vi "xiLIB - LoadFromINI_DIALOG.vi"(6 "IniPath":path=path "C:/Users/Durnek60/Desktop/3DLIB/APP_REQ/APP_FOLDER/Setup/Param.ini", 8 "error in (no error)":errorcluster, 11 "xiCam In":refnum<k24>) -> (0 "error out":errorcluster={"status"=TRUE, "code"=-1, "source"="Parameter file not found at location: \n\nC:\\Users\\Durnek60\\Desktop\\3DLIB\\Resources\\Cam_PRM.ini"}, 3 "xiCam Out":refnum<k24>)   [LabVIEW 2018]
doc: "Dialog based parameter load function."
uses:
  D:/codes labview/VisionLibrariesXimea/xiLib/xiLIB_64bit/xiLIB/xiCamLib/API/x64/xiApi.NETX64.dll
  API/x64/xiApi.NETX64.dll
  xiCam/PRM/PRM/PRM_v2.ctl
  <vilib>/Utility/miscctls.llb/LVRowAndColumnTypeDef.ctl
  <vilib>/Utility/config.llb/NI_LVConfig.lvlib
panel:
  in  "MCL":i32(listbox)=-1
  out "Slide":i32(slide) caption="Loading..." min=0 scale=0.0..91.0
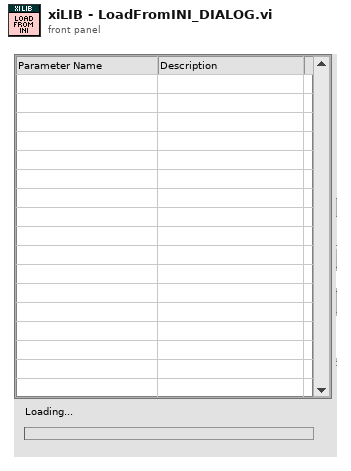
[diagram p1: front panel]
types:
  T1 = typedef "PRM_v2.ctl" = enum16{"ACQ_BUFFER_SIZE", "ACQ_FRAME_BURST_COUNT", "ACQ_TIMING_MODE", "ACQ_TRANSPORT_BUFFER_SIZE", "AE_MAX_LIMIT", "AEAG", "AEAG_LEVEL", "API_VERSION", "AG_MAX_LIMIT", "APPLY_CMS", "AUTO_BANDWIDTH_CALCULATION", "AUTO_WB", "AVAILABLE_BANDWIDTH", "AVAILABLE_BANDWIDTH_MAX", "AVAILABLE_BANDWIDTH_MIN", "BPC", "BUFFER_POLICY", "BUFFERS_QUEUE_SIZE", "CC_MATRIX_00", "CC_MATRIX_01", "CC_MATRIX_02", "CC_MATRIX_03", "CC_MATRIX_10", "CC_MATRIX_11", "CC_MATRIX_12", "CC_MATRIX_13", "CC_MATRIX_20", "CC_MATRIX_21", "CC_MATRIX_22", "CC_MATRIX_23", "CC_MATRIX_30", "CC_MATRIX_31", "CC_MATRIX_32", "CC_MATRIX_33", "CHIP_TEMP", "CMS", "COLOR_FILTER_ARRAY", "COOLING", "DEBOUNCE_EN", "DEBOUNCE_POL", "DEBOUNCE_T0", "DEBOUNCE_T1", "DEBUG_LEVEL", "DEFAULT_CC_MATRIX", "DEVICE_INSTANCE_PATH", "DEVICE_MODEL_ID", "DEVICE_NAME", "DEVICE_SN", "DEVICE_TYPE", "DEVICE_USER_ID", "DOWNSAMPLING", "DOWNSAMPLING_MAX", "DOWNSAMPLING_MIN", "DOWNSAMPLING_TYPE", "DRV_VERSION", "EXP_PRIORITY", "EXPOSURE", "EXPOSURE_DIRECT_UPDATE", "EXPOSURE_MAX", "EXPOSURE_MIN", "FFS_FILE_NAME", "FPGA1_VERSION", "FRAMERATE", "FRAMERATE_MAX", "FRAMERATE_MIN", "FREE_FFS_SIZE", "GAIN", "GAIN_DIRECT_UPDATE", "GAIN_MAX", "GAIN_MIN", "GAMMAC", "GAMMAY", "GPI_LEVEL", "GPI_MODE", "GPI_SELECTOR", "GPI_SELECTOR_MAX", "GPI_SELECTOR_MIN", "GPO_MODE", "GPO_SELECTOR", "GPO_SELECTOR_MAX", "GPO_SELECTOR_MIN", "HDR", "HDR_T1", "HDR_T2", "HEIGHT", "HEIGHT_MAX", "HEIGHT_MIN", "HOUSE_TEMP", "IMAGE_DATA_FORMAT", "IMAGE_IS_COLOR", "INPUT_CMS_PROFILE", "IS_COOLED", "IS_DEVICE_EXIST", "KNEEPOINT1", "KNEEPOINT2", "LED_MODE", "LED_SELECTOR", "LED_SELECTOR_MAX", "LED_SELECTOR_MIN", "LIMIT_BANDWIDTH", "LIMIT_BANDWIDTH_MAX", "LIMIT_BANDWIDTH_MIN", "LUT_EN", "LUT_INDEX", "LUT_INDEX_MAX", "LUT_INDEX_MIN", "LUT_VALUE", "LUT_VALUE_MAX", "LUT_VALUE_MIN", "MANUAL_WB", "MCU1_VERSION", "MCU2_VERSION", "OFFSET_X", "OFFSET_X_MAX", "OFFSET_X_MIN", "OFFSET_Y", "OFFSET_Y_MAX", "OFFSET_Y_MIN", "OUTPUT_CMS_PROFILE", "OUTPUT_DATA_BIT_DEPTH", "OUTPUT_DATA_PACKING", "READ_FILE_FFS", "RECENT_FRAME", "SENSOR_DATA_BIT_DEPTH", "SENSOR_MODE", "SENSOR_TAPS", "SHARPNESS", "SHUTTER_TYPE", "TARGET_TEMP", "TRG_DELAY", "TRG_SELECTOR", "TRG_SOFTWARE", "TRG_SOURCE", "USED_FFS_SIZE", "WB_KB", "WB_KG", "WB_KR", "WIDTH", "WIDTH_MAX", "WIDTH_MIN", "WRITE_FILE_FFS", "ACQ_BUFFER_SIZE_UNIT", "ACQ_TRANSPORT_BUFFER_COMMIT", "AEAG_ROI_HEIGHT", "AEAG_ROI_OFFSET_X", "AEAG_ROU_OFFSET_Y", "AEAG_ROI_WIDTH", "API_CONTEXT_LIST", "BINNING_HORIZONTAL", "BINNING_SELECTOR", "BINNING_VERTICAL", "COLUMN_FPN_CORRECTION", "COUNTER_SELECTOR", "COUNTER_VALUE", "DECIMATION_HORIZONTAL", "DECIMATION_SELECTOR", "DECIMATION_VERTICAL", "DEVICE_ID", "DEVICE_LOCATION_PATH", "DEVICE_MANIFEST", "DEVICE_RESET", "DEVICE_SENS_SN", "EXPOSURE_BURST_COUNT", "FFS_ACCESS_KEY", "GAIN_SELECTOR", "HW_REVISION", "IMAGE_BLACK_LEVEL", "IMAGE_DATA_BIT_DEPTH", "IMAGE_DATA_FORMAT_RGB32_ALPHA", "IMAGE_PAYLOAD_SIZE", "LENS_APERTURE_VALUE", "LENS_FEATURE", "LENS_FEATURE_SELECTOR", "LENS_FOCAL_LENGTH", "LENS_FOCUS_DISTANCE", "LENS_FOCUS_MOVE", "LENS_FOCUS_MOVEMENT_VALUE", "LENS_MODE", "OUTPUT_DATA_PACKING_TYPE", "SENSOR_CLOCK_FREQ_HZ", "SENSOR_CLOCK_FREQ_INDEX", "SENSOR_FEATURE_SELECTOR", "SENSOR_FEATURE_VALUE", "SENSOR_OUTPUT_CHANNEL_COUNT", "TRANSPORT_PIXEL_FORMAT", "TS_RST_MODE", "TS_RST_SOURCE"}
  T2 = typedef "LVRowAndColumnTypeDef.ctl" = cluster{"Row":i32, "Column":i32}
  T3 = typedef "NI_LVConfig.lvlib/Config Data RefNum.ctl" = refnum<k1>
  T4 = typedef "xiLIB - PRM_Load_Result.ctl" = enum16{"SUCCESS", "ERROR", "WARNING - Not Valid Parameter", "WARNING - Get Parameter"}
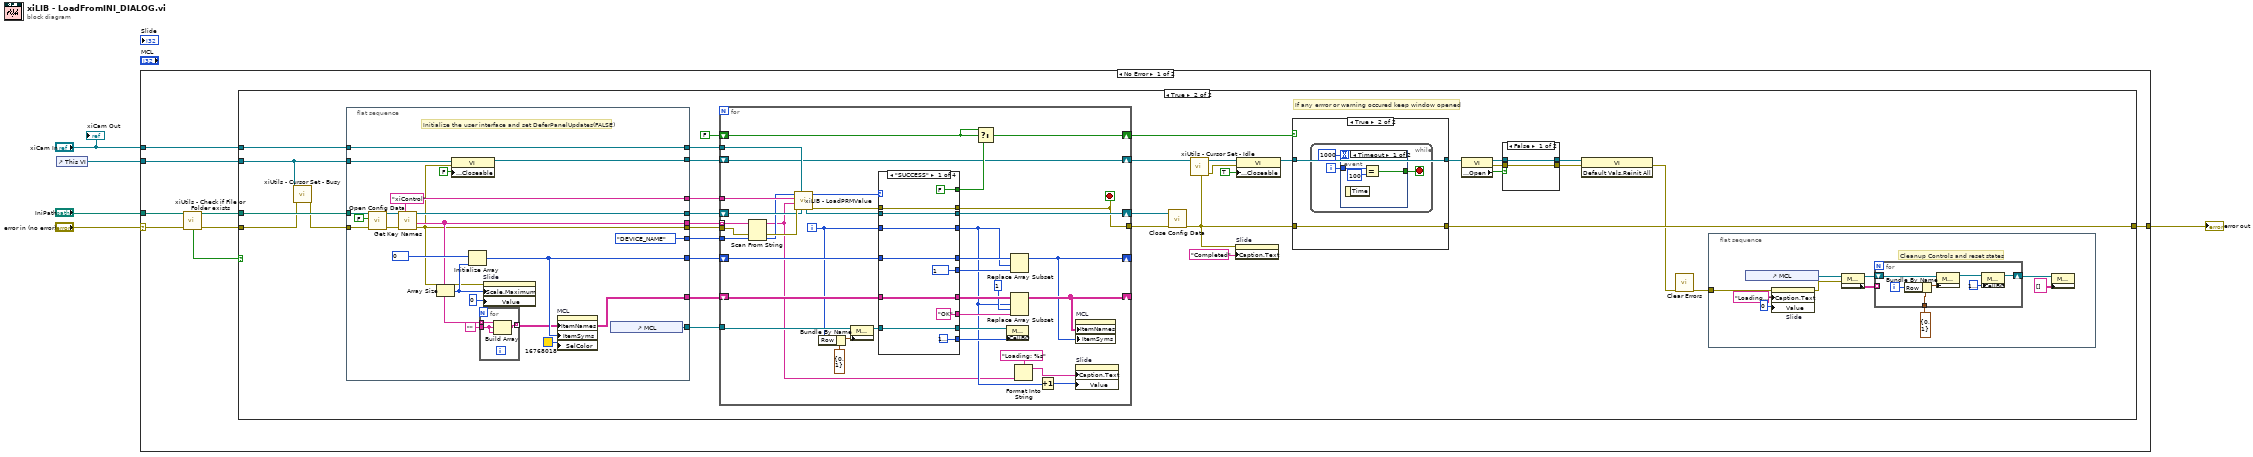
[diagram p0: block diagram]
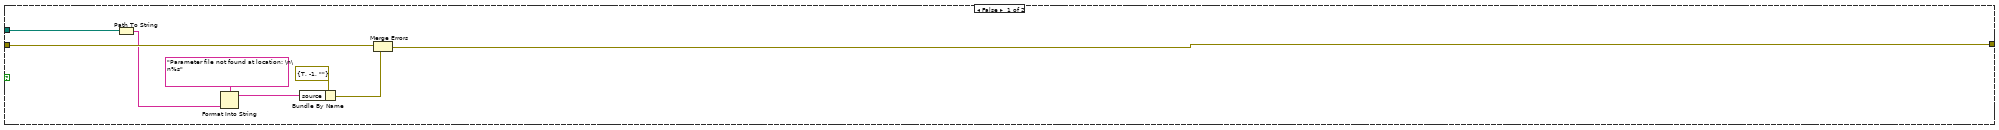
[diagram p2: hidden frame]
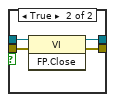
[diagram p3: hidden frame]
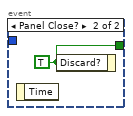
[diagram p5: hidden frame]
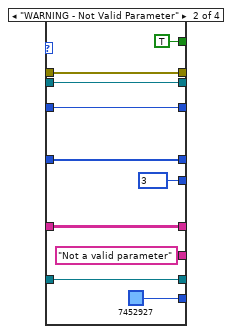
[diagram p6: hidden frame]
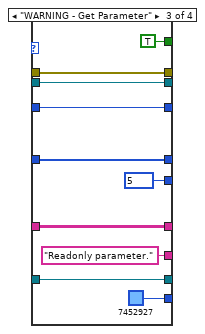
[diagram p7: hidden frame]
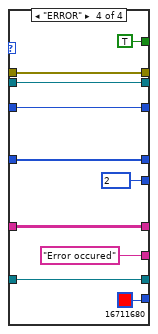
[diagram p8: hidden frame]
diagram:
  n1 = control-ref of="This VI"() -> (w1:refnum<vi>)
  n2 = case shown="No Error" "error in (no error)" {
    selector: "error in (no error)" -> [w10 w192]
    tunnel: [w13 w192] -> w4
    tunnel: "IniPath" -> [w11 _]
    tunnel: "xiCam In" -> [w12 _]
    tunnel: w1 -> [w6 _]
    frame No Error {
      n3 = call "xiUtils - Check if File or Folder exists.vi"("error in (no error)"=w10, "path"=w11) -> ("error out"=w9:errorcluster, "file or folder exists?"=w7:bool, "dup path"=w8:path)  [unwired: 7 in]
      n4 = case shown="True" w7 {
        tunnel: [w20 w44] -> w13
        tunnel: w12 -> [_ w40]
        tunnel: w9 -> [w21 w36]
        tunnel: w8 -> [w19 w38]
        tunnel: w6 -> [_ w37]
        frame False {
          n5 = Path To String(path=w19) -> (string=w17:string)
          n6 = Format Into String(format string="Parameter file not found at location: \n\n%s" ("source"), w17) -> (resulting string=w15:string)  [unwired: 2 in, 1 out]
          n7 = Bundle By Name(cluster=errorcluster {"status"=TRUE, "code"=-1, "source"=""} ("error in"), "source"=w15) -> (w14:errorcluster)
          n8 = Merge Errors(w21, w14) -> (w20:errorcluster)
        }
        frame True {
          # "If any errror or warning occured keep window opened"
          n9 = call "xiUtils - Cursor Set - Busy.vi"("error in (no error)"=w36, "VI reference (Top Level VI)"=w37) -> ("error out"=w35:errorcluster)  [unwired: 8 in, 1 out]
          n10 = flat-sequence {
            tunnel: w38 -> [w83]
            tunnel: w35 -> [w81]
            tunnel: [w78] -> w55
            tunnel: [PRM_v2."DEVICE_NAME" ("PRM")] -> w54
            tunnel: [w76] -> w53
            tunnel: [w71] -> w49
            tunnel: [w70] -> w48
            tunnel: [w68] -> w47
            tunnel: [w67] -> w46
            tunnel: [w66] -> w45
            tunnel: w40 -> [w65]
            tunnel: [w65] -> w39
            tunnel: w37 -> [w63]
            tunnel: [w62] -> w33
            frame #0 {
              w76 = "xiControl" ("section")
              # "Initialize the user interface and set DeferPanelUpdates(FALSE)"
              n11 = call <vilib>:"Open Config Data.vi"("error in (no error)"=w81, "create file if necessary (T)"=FALSE, "configuration file path"=w83) -> ("error out"=w79:errorcluster, "refnum"=w80:T3)  [unwired: 6 in, 1 out]
              n12 = call <vilib>:"Get Key Names.vi"("section"=w76, "error in (no error)"=w79, "refnum"=w80) -> ("error out"=w67:errorcluster, "key names"=w71:string[], "refnum out"=w78:T3)  [unwired: 5 in, 1 out]
              n13 = Array Size(array=w71) -> (size(s)=w72:i32)
              n14 = property class="VI"(reference=w63, error in=w67, "Front Panel.Closeable"=FALSE ("Front Panel Window:Closeable")) -> (reference out=w62:refnum<vi>)  [unwired: 1 out]
              n15 = Initialize Array(0, w72) -> (w70:i32[])
              n16 = for {
                tunnel: w71 -> [w86] mode=indexing
                tunnel: [w85] -> w68 mode=indexing
                tunnel: "" -> [w84]
                n17 = Build Array(w86, w84, w84) -> (w85:string[])
              }
              n18 = property on="Slide" class="Slide (strict)"(error in=w67, "Scale.Maximum"=w72, "Value"=0 ("Slide")) -> ()  [unwired: 1 in, 2 out]
              n19 = property on="MCL" class="MCListbox (strict)"("ItemNames"=w68, "ItemSyms"=w70, "SelColor"=u32 16768018) -> ()  [unwired: 2 in, 2 out]
              n20 = control-ref of="MCL"() -> (w66:refnum<vi>)
            }
          }
          n21 = for {
            shift-right: [w139] -> w52
            shift-left: w55 -> [w149]
            tunnel: w49 -> [w117] mode=indexing
            tunnel: w54 -> [w151]
            tunnel: w46 -> [w148]
            tunnel: w53 -> [w147]
            shift-right: [w122] -> _
            shift-left: w48 -> [w138]
            tunnel: w39 -> [w143]
            shift-right: [w145] -> w50
            shift-left: FALSE -> [w146]
            shift-right: [w123] -> _
            shift-left: w47 -> [w135]
            tunnel: w45 -> [w129]
            tunnel: [w124] -> w42
            shift-right: [w115] -> w32
            shift-left: w33 -> [w115]
            i -> [w128]
            stop <- w124 stop-if-true
            n22 = Scan From String(input string=w117, error in=w148, default 1=w151) -> (error out=w150:errorcluster, output 1=w144:T1)  [unwired: 2 in, 2 out]
            n23 = call "xiLIB - LoadPRMValue.vi"("INI Refnum"=w149, "xiCam In"=w143, "error in (no error)"=w150, "key"=w117, "section"=w147, "PRM"=w144) -> ("error out"=w141:errorcluster, "Load_Result"=w142:T4, "INI Refnum out"=w140:T3)  [unwired: 3 in]
            n24 = Bundle By Name(cluster=T2 {"Row"=0, "Column"=1} ("Active Cell:Active Cell"), "Row"=w128) -> (w130:T2)
            n25 = property class="MCListbox (strict)"(reference=w129, "ActiveCell"=w130) -> (reference out=w127:refnum<vi>)  [unwired: 1 in, 1 out]
            n26 = case shown="\"SUCCESS\"" w142 {
              tunnel: w141 -> [w160 w170 w180 w190]
              tunnel: w140 -> [w161 w171 w181 w191]
              tunnel: [w161 w171 w181 w191] -> w139
              tunnel: [w160 w170 w180 w190] -> w124
              tunnel: w128 -> [w157 w167 w177 w187]
              tunnel: w138 -> [w159 w169 w179 w189]
              tunnel: [w159 w169 w179 w189] -> w137
              tunnel: [1 3 5 2] -> w136
              tunnel: [w157 w167 w177 w187] -> w118
              tunnel: w135 -> [w156 w166 w176 w186]
              tunnel: [w156 w166 w176 w186] -> w134
              tunnel: ["OK" "Not a valid parameter" "Readonly parameter." "Error occured"] -> w132
              tunnel: w127 -> [w155 w164 w173 w184]
              tunnel: [w155 w164 w173 w184] -> w126
              tunnel: [u32 16777233 ("Color Box") u32 7452927 u32 7452927 u32 16711680] -> w125
              tunnel: [FALSE TRUE TRUE TRUE] -> w116
              frame "SUCCESS" {
              }
              frame "WARNING - Not Valid Parameter" {
              }
              frame "WARNING - Get Parameter" {
              }
              frame "ERROR" {
              }
            }
            n27 = Select(t=w146, s=w146, f=w116) -> (s? t:f=w145:bool)
            n28 = property class="MCListbox (strict)"(reference=w126, "CellBG"=w125) -> ()  [unwired: 1 in, 2 out]
            n29 = Replace Array Subset(array=w137, new element=w136, index=w118) -> (w122:i32[])
            n30 = Replace Array Subset(array=w134, new element=w132, index (row)=w118, index (col)=1) -> (w123:string[][])
            n31 = Format Into String(format string="Loading: %s", w117) -> (resulting string=w119:string)  [unwired: 2 in, 1 out]
            n32 = Increment(x=w118) -> (x+1=w121:i32)
            n33 = property on="Slide" class="Slide (strict)"("Caption.Text"=w119, "Value"=w121) -> ()  [unwired: 2 in, 2 out]
            n34 = property on="MCL" class="MCListbox (strict)"("ItemNames"=w123, "ItemSyms"=w122) -> ()  [unwired: 2 in, 2 out]
          }
          n35 = call <vilib>:"Close Config Data.vi"("error in (no error)"=w42, "refnum"=w52) -> ("error out"=w31:errorcluster)  [unwired: 8 in, 1 out]
          n36 = call "xiUtils - Cursor Set - Idle.vi"("error in (no error)"=w31, "VI reference (Top Level VI)"=w32) -> ("error out"=w30:errorcluster)  [unwired: 9 in]
          n37 = property on="Slide" class="Slide (strict)"(error in=w31, "Caption.Text"="Completed" ("format string")) -> ()  [unwired: 1 in, 2 out]
          n38 = property class="VI"(reference=w32, error in=w30, "Front Panel.Closeable"=TRUE ("Front Panel Window:Closeable")) -> (reference out=w26:refnum<vi>)  [unwired: 1 out]
          n39 = case shown="True" w50 {
            tunnel: w31 -> [w105 w107]
            tunnel: [w105 w107] -> w44
            tunnel: w26 -> [w104 w106]
            tunnel: [w104 w106] -> w25
            frame False {
              # "Do nothing, every parameter loaded"
            }
            frame True {
              n40 = while {
                i -> [w108]
                stop <- w110 stop-if-true
                n41 = event shown="[0] Timeout" {
                  selector: _ -> [_ _]
                  dyn-events: _ -> [_ _]
                  timeout: 1000 -> [_ _]
                  tunnel: [w111 w114] -> w110
                  tunnel: w108 -> [w113 _]
                  event Timeout {
                    n42 = event-data() -> ()  [unwired: 1 in, 1 out]
                    n43 = Equal?(x=w113, y=100) -> (x = y?=w111:bool)
                  }
                  event Panel Close? {
                    w114 = TRUE
                    n44 = event-data() -> ()  [unwired: 1 in, 1 out]
                    n45 = event-data("Discard?"=w114) -> ()  [unwired: 1 in, 1 out]
                  }
                }
              }
            }
          }
          n46 = property class="VI"(reference=w25) -> (reference out=w28:refnum<vi>, error out=w29:errorcluster, "Front Panel.Open"=w27:bool)  [unwired: 1 in]
          n47 = case shown="False" w27 {
            tunnel: [w57 w61] -> w23
            tunnel: w29 -> [w57 w60]
            tunnel: w28 -> [w56 w59]
            tunnel: [w56 w58] -> w24
            frame False {
            }
            frame True {
              n48 = invoke class="VI" method="FP.Close"(reference=w59, error in=w60) -> (reference out=w58:refnum<vi>, error out=w61:errorcluster)  [unwired: 1 in, 1 out]
            }
          }
          n49 = invoke class="VI" method="Default Vals.Reinit All"(reference=w24, error in=w23) -> (error out=w22:errorcluster)  [unwired: 1 in, 2 out]
          n50 = call <vilib>:"Clear Errors.vi"("error in (no error)"=w22) -> ("error out"=w41:errorcluster)  [unwired: 5 in, 1 out]
          n51 = flat-sequence {
            tunnel: w41 -> [w90]
            frame #0 {
              # "Cleanup Controls and reset states"
              n52 = control-ref of="MCL"() -> (w96:refnum<vi>)
              n53 = property on="Slide" class="Slide (strict)"(error in=w90, "Caption.Text"="Loading...", "Value"=0 ("Slide")) -> (error out=w87:errorcluster)  [unwired: 1 in, 1 out]
              n54 = property class="MCListbox (strict)"(reference=w96, error in=w87) -> (reference out=w94:refnum<vi>, "ItemNames"=w95:string[][])  [unwired: 1 out]
              n55 = for {
                tunnel: w95 -> [_] mode=indexing
                shift-right: [w98] -> w93
                shift-left: w94 -> [w102]
                tunnel: T2 {"Row"=0, "Column"=1} ("Active Cell:Active Cell") -> [w97]
                i -> [w101]
                n56 = Bundle By Name(cluster=w97, "Row"=w101) -> (w103:T2)
                n57 = property class="MCListbox (strict)"(reference=w102, "ActiveCell"=w103) -> (reference out=w100:refnum<vi>)  [unwired: 1 in, 1 out]
                n58 = property class="MCListbox (strict)"(reference=w100, "CellBG"=u32 16777233 ("Color Box")) -> (reference out=w98:refnum<vi>)  [unwired: 1 in, 1 out]
              }
              n59 = property class="MCListbox (strict)"(reference=w93, "ItemNames"=string[][] [] ("Item Names")) -> ()  [unwired: 1 in, 2 out]
            }
          }
        }
      }
    }
    frame Error {
    }
  }
  "error out" <- w4
  "xiCam Out" <- "xiCam In"
